vi "Current Match Control.vi"(9 "New Phase":enum16{"Practice", "Ranking"}(ring), 10 "New Match":u16, 11 "Mode":T1(ring)) -> (1 "Current Phase":enum16{"Practice", "Ranking"}(ring), 2 "Current Match":u16)   [LabVIEW 2013]
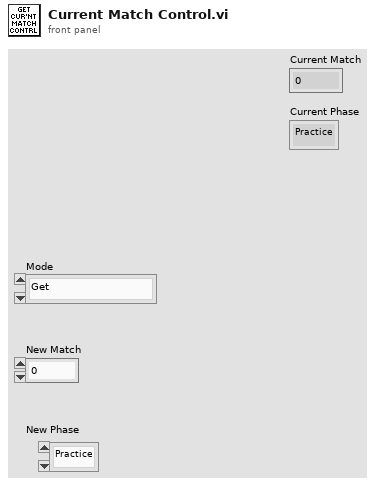
[diagram p1: front panel]
types:
  T1 = enum16{"Get", "Increment", "Decrement", "Set Match", "Set Phase"}
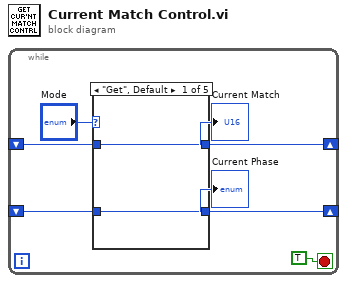
[diagram p0: block diagram]
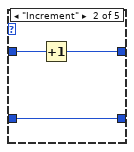
[diagram p2: hidden frame]
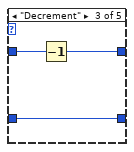
[diagram p3: hidden frame]
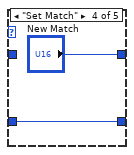
[diagram p4: hidden frame]
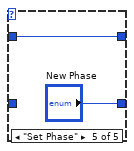
[diagram p5: hidden frame]
diagram:
  n1 = while {
    shift-right: [w4] -> _
    shift-left: _ -> [w3]
    shift-right: [w2] -> _
    shift-left: _ -> [w1]
    stop <- TRUE stop-if-true
    n2 = case shown="\"Get\", Default" "Mode" {
      tunnel: [w8 w11 w13 "New Match" w17] -> w4
      tunnel: w3 -> [w8 w10 w14 _ w17]
      tunnel: [w7 w9 w12 w15 "New Phase"] -> w2
      tunnel: w1 -> [w7 w9 w12 w15 _]
      frame "Get", Default {
      }
      frame "Increment" {
        n3 = Increment(x=w10) -> (x+1=w11:u16)
      }
      frame "Decrement" {
        n4 = Decrement(x=w14) -> (x-1=w13:u16)
      }
      frame "Set Match" {
      }
      frame "Set Phase" {
      }
    }
    "Current Match" <- w4
    "Current Phase" <- w2
  }
